vi "DropTag__slk_mt.vi"(8 "error in (no error)":errorcluster, 11 "tree view in":refnum<class "TreeView__slk_mt.lvclass">) -> (0 "error out":errorcluster, 3 "tree view out":refnum<class "TreeView__slk_mt.lvclass">)   [LabVIEW 2014, in "Lazyboots Menu Tool.lvlib" / "TreeView__slk_mt.lvclass"]
doc: "Drops a tag."
uses:
  TreeView__slk_mt.lvclass
  TreeView__slk_mt.lvclass/TreeView__slk_mt.ctl
panel:
  # "DropTag__slk_mt.vi\nDrops a tag.\n\nNOTICE -- YOU MUST LEAVE THIS NOTICE IN PLACE.\n\nCopyright (c) 2011, LIANG LIU Shawn.Liu.cn@gmail.com\nAll rights reserved.\n\nRedistribution and use in source and binary forms, with or without modification, are permitted provided that the following conditions are met:\n-Redistributions of source code must retain the above copyright notice, this list of conditions and the following disclaimer.\n-Redistributions in binary form must reproduce the above copyright notice, this list of conditions and the following disclaimer in the documentation and/or other materials provided with the distribution.\n-Neither the name of the eLp nor the names of its contributors may be used to endorse or promote products derived from this software without specific prior written permission.\n\nTHIS SOFTWARE IS PROVIDED BY THE COPYRIGHT HOLDERS AND CONTRIBUTORS \"AS IS\" AND ANY EXPRESS OR IMPLIED WARRANTIES, INCLUDING, BUT NOT LIMITED TO, THE IMPLIED WARRANTIES OF MERCHANTABILITY AND FITNESS FOR A PARTICULAR PURPOSE ARE DISCLAIMED. IN NO EVENT SHALL THE COPYRIGHT HOLDER OR CONTRIBUTORS BE LIABLE FOR ANY DIRECT, INDIRECT, INCIDENTAL, SPECIAL, EXEMPLARY, OR CONSEQUENTIAL DAMAGES (INCLUDING, BUT NOT LIMITED TO, PROCUREMENT OF SUBSTITUTE GOODS OR SERVICES; LOSS OF USE, DATA, OR PROFITS; OR BUSINESS INTERRUPTION) HOWEVER CAUSED AND ON ANY THEORY OF LIABILITY, WHETHER IN CONTRACT, STRICT LIABILITY, OR TORT (INCLUDING NEGLIGENCE OR OTHERWISE) ARISING IN ANY WAY OUT OF THE USE OF THIS SOFTWARE, EVEN IF ADVISED OF THE POSSIBILITY OF SUCH DAMAGE."
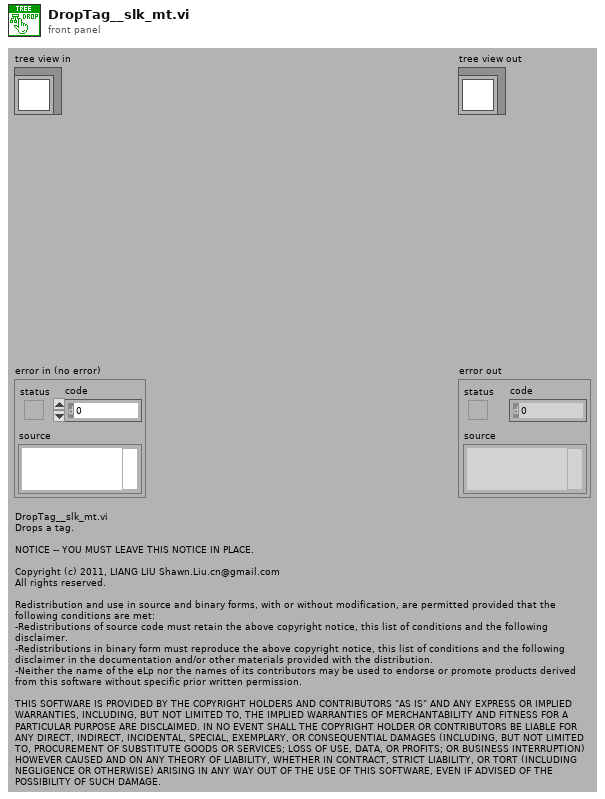
[diagram p1: front panel]
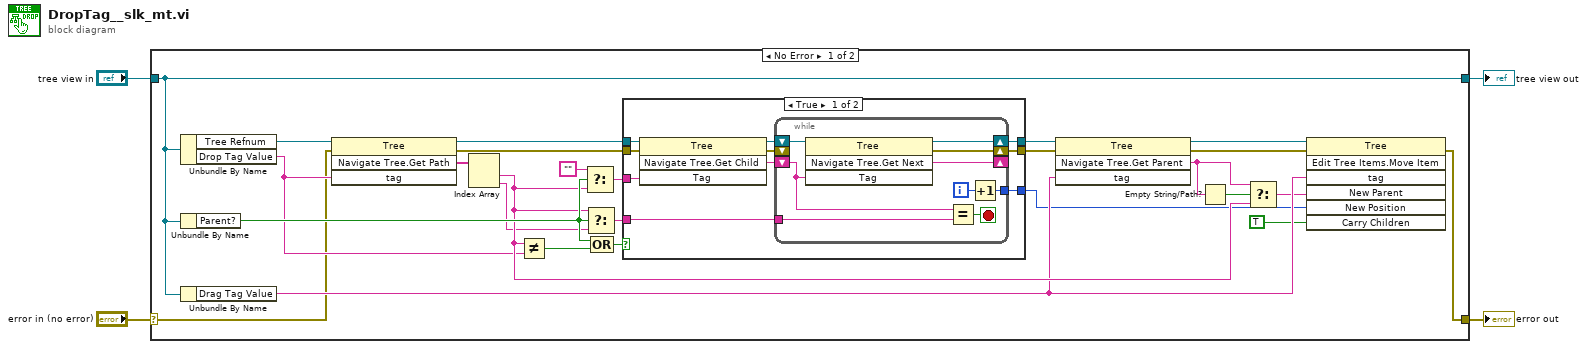
[diagram p0: block diagram]
diagram:
  n1 = case shown="No Error" "error in (no error)" {
    selector: "error in (no error)" -> [w5 w53]
    tunnel: [w6 w53] -> w3
    tunnel: [w13 w52] -> w1
    tunnel: "tree view in" -> [w13 w52]
    frame No Error {
      n2 = Unbundle By Name(w13) -> ("Tree Refnum"=w27:refnum<vi>, "Drop Tag Value"=w26:string)
      n3 = Unbundle By Name(w13) -> ("Parent?"=w30:bool)
      n4 = Unbundle By Name(w13) -> ("Drag Tag Value"=w21:string)
      n5 = invoke class="Tree" method="Navigate Tree.Get Path"(reference=w27, error in=w5, "tag"=w26) -> (reference out=w18:refnum<vi>, error out=w17:errorcluster, "Navigate Tree:Get Path"=w19:string[])  [unwired: 1 in, 1 out]
      n6 = Index Array(array=w19) -> (element #1=w28:string, element #2=w24:string)  [unwired: 2 in]
      n7 = Not Equal?(x=w28, y=w26) -> (x != y?=w20:bool)
      n8 = Select(t="", s=w30, f=w28) -> (s? t:f=w22:string)
      n9 = Select(t=w28, s=w30, f=w24) -> (s? t:f=w25:string)
      n10 = Compound Arithmetic op=OR(w30, w20) -> (w29:bool)
      n11 = case shown="True" w29 {
        tunnel: w22 -> [w40 _]
        tunnel: w18 -> [w39 w51]
        tunnel: w17 -> [w38 w50]
        tunnel: w25 -> [w34 _]
        tunnel: [w33 _] -> w15
        tunnel: [w32 w51] -> w14
        tunnel: [w31 w50] -> w16
        frame True {
          n12 = invoke class="Tree" method="Navigate Tree.Get Child"(reference=w39, error in=w38, "Tag"=w40) -> (reference out=w37:refnum<vi>, error out=w36:errorcluster, "Navigate Tree:Get Child"=w35:string)  [unwired: 1 in, 1 out]
          n13 = while {
            shift-right: [w45] -> w31
            shift-left: w36 -> [_]
            shift-right: [w48] -> _
            shift-left: w35 -> [w43]
            tunnel: w34 -> [w47]
            shift-right: [w46] -> w32
            shift-left: w37 -> [w49]
            tunnel: [w41] -> w33
            i -> [w42]
            stop <- w44 stop-if-true
            n14 = invoke class="Tree" method="Navigate Tree.Get Next"(reference=w49, "Tag"=w43) -> (reference out=w46:refnum<vi>, error out=w45:errorcluster, "Navigate Tree:Get Next Item"=w48:string)  [unwired: 2 in, 1 out]
            n15 = Equal?(x=w43, y=w47) -> (x = y?=w44:bool)
            n16 = Increment(x=w42) -> (x+1=w41:i32)
          }
        }
        frame False {
        }
      }
      n17 = invoke class="Tree" method="Navigate Tree.Get Parent"(reference=w14, error in=w16, "tag"=w21) -> (reference out=w11:refnum<vi>, error out=w10:errorcluster, "Navigate Tree:Get Parent"=w7:string)  [unwired: 1 in, 1 out]
      n18 = Empty String/Path?(string/path=w7) -> (empty?=w8:bool)
      n19 = Select(t=w7, s=w8, f=w28) -> (s? t:f=w9:string)
      n20 = invoke class="Tree" method="Edit Tree Items.Move Item"(reference=w11, error in=w10, "tag"=w21, "New Parent"=w9, "New Position"=w15, "Carry Children"=TRUE ("Carry Children?")) -> (error out=w6:errorcluster)  [unwired: 1 in, 6 out]
    }
    frame Error {
    }
  }
  "error out" <- w3
  "tree view out" <- w1
